vi "dfd_Check Num of MRate Filter.vi"(8 "error in (no error)":errorcluster, 11 "#MRate in":i32) -> (0 "error out":errorcluster, 3 "#MRate out":i32)   [LabVIEW 2017, in "NI_DigFilterLicensed.lvlib"]
uses:
  <vilib>/addons/Digital Filter Design/NI_DigFilterLicensed.lvlib
  <vilib>/addons/Digital Filter Design/_Misc.llb/dfd_Error Handlers (Single).vi
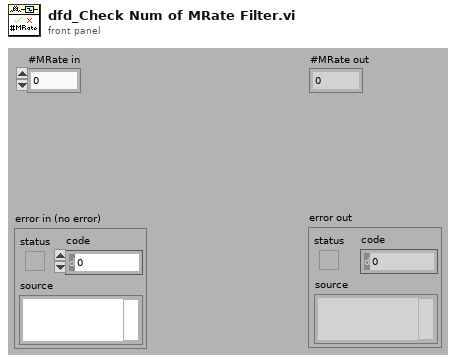
[diagram p1: front panel]
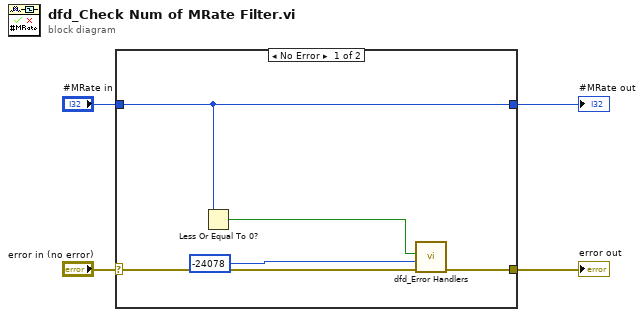
[diagram p0: block diagram]
diagram:
  n1 = case shown="No Error" "error in (no error)" {
    selector: "error in (no error)" -> [w5 w10]
    tunnel: "#MRate in" -> [w9 w11]
    tunnel: [w9 w11] -> w2
    tunnel: [w8 w10] -> w1
    frame No Error {
      n2 = Less Or Equal To 0?(x=w9) -> (x <= 0?=w6:bool)
      n3 = call-poly <vilib>:"dfd_Error Handlers.vi"("error in (no error)"=w5, "error code"=-24078 ("ERR_#MRATE_EQ ZERO"), "condition failed?"=w6) -> ("error out"=w8:errorcluster)  [unwired: 8 out]
    }
    frame Error {
    }
  }
  "error out" <- w1
  "#MRate out" <- w2
